vi "fileio.vi"() -> ()   [LabVIEW 2018]
panel:
  out "Signals":dynamicdata(graph)
  out "Dynamic Data Type":dynamicdata(graph)
  out "text":string
  in  "file path (use dialog) 2":path
  out "cancelled":bool
  in  "file path (use dialog)":path
  # "Escrever no arquivo"
  # "Ler o arquivo"
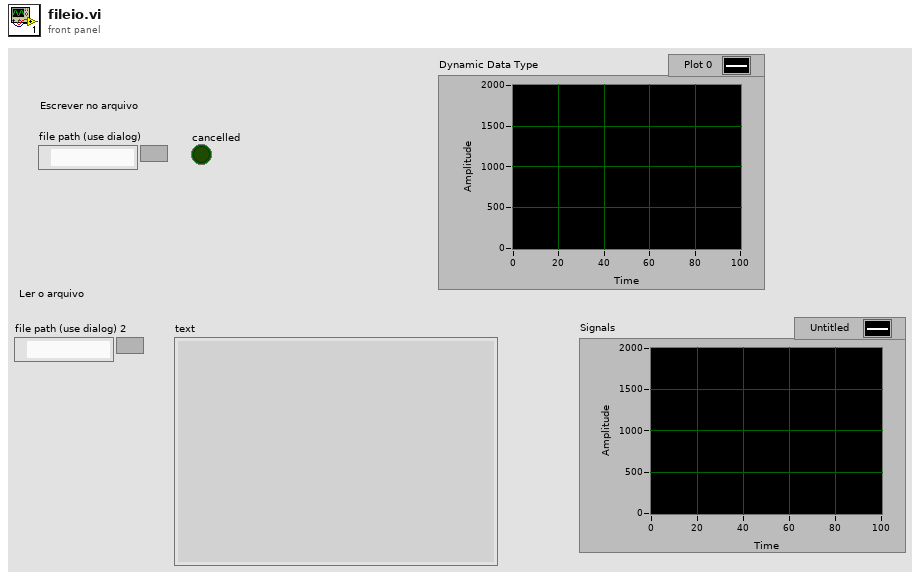
[diagram p1: front panel]
types:
  T1 = enum16{"open", "replace", "create", "open or create", "replace or create", "replace or create with confirmation"}
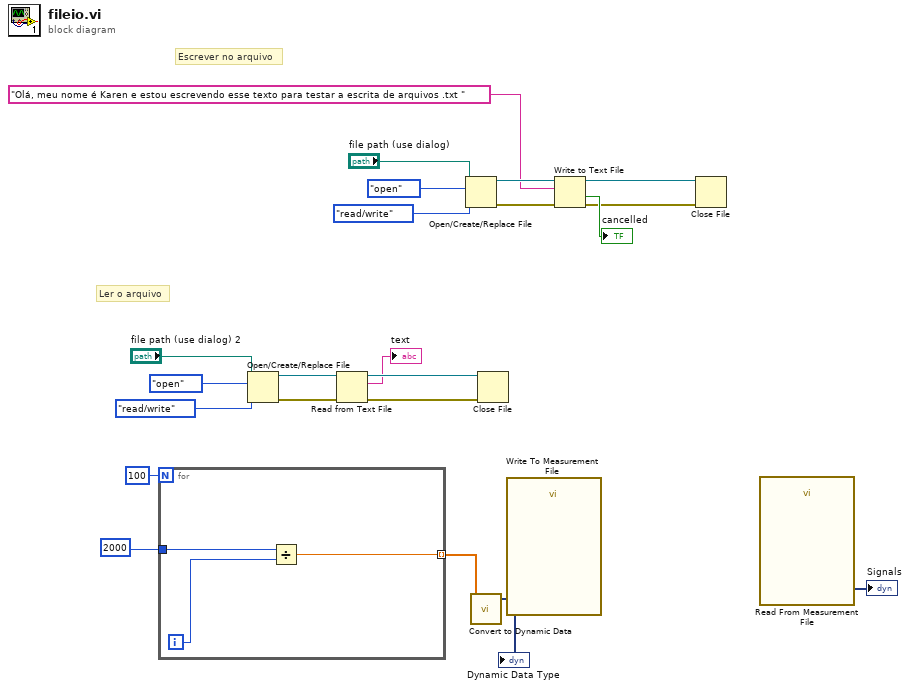
[diagram p0: block diagram]
diagram:
  # "Ler o arquivo"
  # "Escrever no arquivo"
  n1 = for {
    N: 100 -> [_]
    tunnel: 2000 -> [w24]
    tunnel: [w23] -> w3 mode=indexing
    i -> [w25]
    n2 = Divide(x=w24, y=w25) -> (x/y=w23:dbl)
  }
  n3 = Open/Create/Replace File(file path (use dialog)="file path (use dialog) 2", operation (0:open)=T1."open", access (0:read/write)=enum16{"read/write", "read-only", "write-only"}."read/write") -> (refnum out=w13:refnum<file>, error out=w12:errorcluster)  [unwired: 3 in, 1 out]
  n4 = Read from Text File(file (use dialog)=w13, error in=w12) -> (refnum out=w8:refnum<file>, text=→"text":string, error out=w7:errorcluster)  [unwired: 2 in, 1 out]
  n5 = Open/Create/Replace File(file path (use dialog)="file path (use dialog)", operation (0:open)=T1."open", access (0:read/write)=enum16{"read/write", "read-only", "write-only"}."read/write") -> (refnum out=w22:refnum<file>, error out=w21:errorcluster)  [unwired: 3 in, 1 out]
  n6 = call "Convert to Dynamic Data"("Array"=w3) -> ("Dynamic Data Type"=w2:dynamicdata)  [unwired: 3 in]
  "Dynamic Data Type" <- w2
  n7 = Close File(refnum=w8, error in=w7) -> ()  [unwired: 2 out]
  n8 = call "Write To Measurement File"("Signals"=w2) -> ()  [unwired: 16 in, 3 out]
  n9 = Write to Text File(file (use dialog)=w22, text="Olá, meu nome é Karen e estou escrevendo esse texto para testar a escrita de arquivos .txt ", error in=w21) -> (refnum out=w16:refnum<file>, cancelled=→"cancelled":bool, error out=w14:errorcluster)  [unwired: 1 in]
  n10 = Close File(refnum=w16, error in=w14) -> ()  [unwired: 2 out]
  n11 = call "Read From Measurement File"() -> ("Signals"=→"Signals":dynamicdata)  [unwired: 6 in, 5 out]
